vi "n regulation2.vi"(8 "error in (no error)":errorcluster, 9 "fmin":dbl, 10 "fmax":dbl, 11 "n":u16) -> (0 "error out":errorcluster)   [LabVIEW 2015, in "SCANalone4x64.lvlib"]
doc: "__declspec(dllimport) void __stdcall n_regulation2(unsigned short n, double fmax, double fmin);"
uses:
  <userlib>/SCANalone4x64/SCANalone4x64.lvlib
  <userlib>/SCANalone4x64/SCANalone4x64.dll
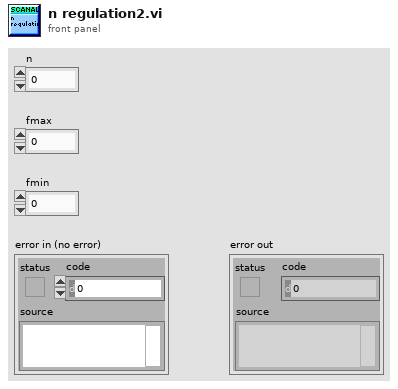
[diagram p1: front panel]
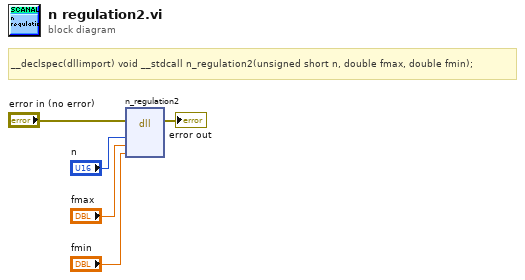
[diagram p0: block diagram]
diagram:
  # "__declspec(dllimport) void __stdcall n_regulation2(unsigned short n, double fmax, double fmin);"
  n1 = dll-call lib="C:/Program Files/National Instruments/LabVIEW 2015/user.lib/SCANalone4x64/SCANalone4x64.*" fn="n_regulation2"(error in="error in (no error)", "n"="n", "fmax"="fmax", "fmin"="fmin") -> (error out=→"error out":errorcluster)  [unwired: 6 in, 1 out]
